vi "message_sendReply.vi"(0 "Host_Reference":refnum<class "HGF_Reference.lvclass">, 1 "MoAgSy_Message":refnum<class "MoAgSy_Message.lvclass">, 2 "timeout in ms (-1)":i32=-1, 5 "error in (no error)":errorcluster, 6 "Message":string, 8 "message":T1(ring), 9 "Message Type":enum16{"error Reply", "reply", "PublicKey"}(ring)) -> (14 "dup Host_Reference":refnum<class "HGF_Reference.lvclass">, 19 "error out":errorcluster)   [LabVIEW 2009, in "MoAgSy.lvlib" / "MoAgSy_Host.lvclass"]
doc: "<B>public</B> VI sends reply from referenced Host to an incoming message.\n<B> still in progress, only SV available</B>\n\nF.Berck@gsi.de\nGSI Darmstadt 2009"
uses:
  MoAgSy_Host.lvclass
  HGF_BaseClasses/HGF_Reference/HGF_Reference.lvclass
  MoAgSy_Message/MoAgSy_Message.lvclass
  MoAgSy_Factory/MoAgSy_Factory.lvclass
  HGF_BaseClasses/HGF_Factory/HGF_Factory.lvclass
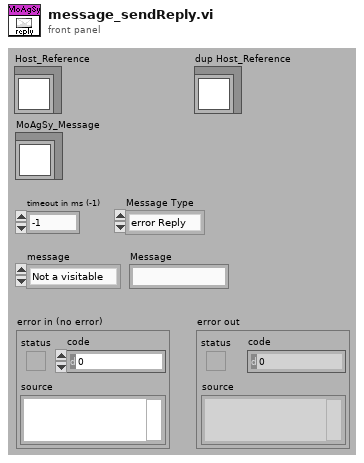
[diagram p1: front panel]
types:
  T1 = enum16{"Not a visitable", "Agent blacklisted", "Host full", "ok", "Class Unknown"}
  T2 = cluster{"Host Name":string, "Maximum number of running Agents":i16, "ID":string}
  T3 = cluster{"Host Variable":refnum<k21>, "Agent_Event (Monitor Event)":refnum<class "HGF_Event.lvclass">, "Host_Event (Monitor Event)":refnum<class "HGF_Event.lvclass">, "DSCException":refnum<class "HGF_TriggeredEvent.lvclass">, "MoAgSy_DSCThreadPool":refnum<class "HGF_Reference.lvclass">, "ManagerEvent":refnum<class "HGF_Event.lvclass">, "DSCDestination":refnum<class "HGF_TriggeredEvent.lvclass">}
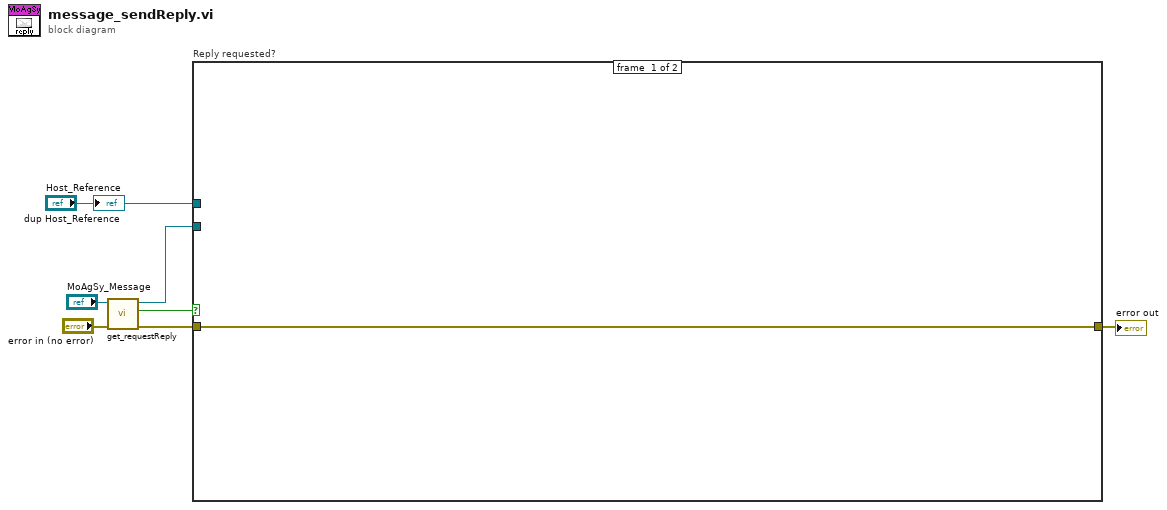
[diagram p0: block diagram]
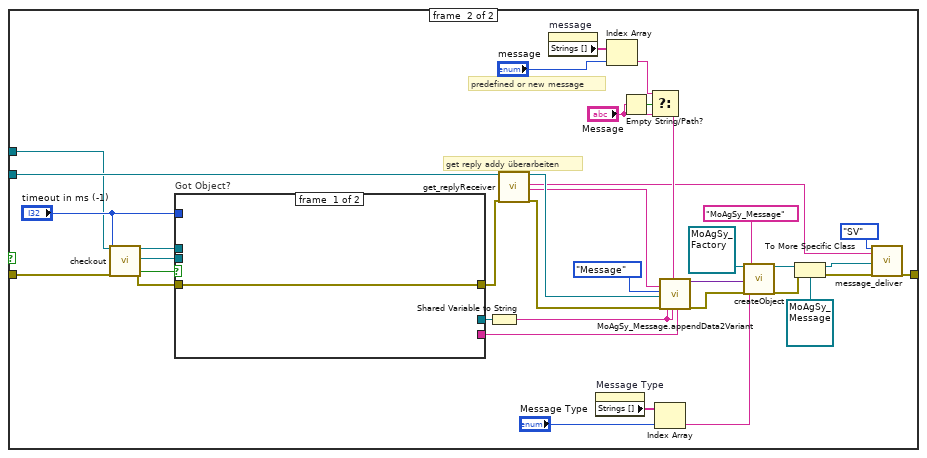
[diagram p2: hidden frame]
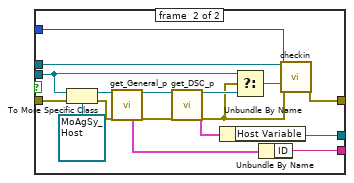
[diagram p3: hidden frame]
diagram:
  n1 = call "get_requestReply.vi"("error in (no error)"="error in (no error)", "MoAgSy_Message.lvclass in"="MoAgSy_Message") -> ("error out"=w2:errorcluster, "request reply"=w4:bool, "MoAgSy_Message.lvclass out"=w5:refnum<class "MoAgSy_Message.lvclass">)  [unwired: 7 out]
  n2 = case "Reply requested?" shown="True" w4 {
    tunnel: w5 -> [_ w35]
    tunnel: [w8 w18] -> w7
    tunnel: w2 -> [w8 w17]
    tunnel: "Host_Reference" -> [_ w16]
    frame #0 {
    }
    frame #1 {
      # "predefined or new message"
      # "get reply addy überarbeiten"
      n3 = call "checkout.vi"("HGF_Reference"=w16, "timeout in ms (-1)"="timeout in ms (-1)", "error in (no error)"=w17) -> ("dup HGF_Reference"=w41:refnum<class "HGF_Reference.lvclass">, "Object"=w43:refnum<class>, "got object?"=w42:bool, "error out"=w44:errorcluster)  [unwired: 13 out]
      n4 = case "Got Object?" shown="True" w42 {
        tunnel: w43 -> [_ w57]
        tunnel: w41 -> [_ w62]
        tunnel: "timeout in ms (-1)" -> [_ w61]
        tunnel: [w46 w60] -> w33
        tunnel: w44 -> [w46 w59]
        tunnel: [_ w55] -> w14
        tunnel: [_ w53] -> w24
        frame #0 {
        }
        frame #1 {
          n5 = To More Specific Class(target class=refnum<class "MoAgSy_Host.lvclass"> refnum ("MoAgSy.lvlib:MoAgSy_Host.lvclass"), reference=w57, error in=w59) -> (specific class reference=w52:refnum<class "MoAgSy_Host.lvclass">, error out=w50:errorcluster)
          n6 = call "get_General_p.vi"("MoAgSy_Host"=w52, "error in (no error)"=w50) -> ("dup MoAgSy_Host"=w48:refnum<class "MoAgSy_Host.lvclass">, "General"=w56:T2, "error out"=w49:errorcluster)  [unwired: 15 out]
          n7 = call "get_DSC_p.vi"("MoAgSy_Host"=w48, "error in (no error)"=w49) -> ("dup MoAgSy_Host"=w51:refnum<class "MoAgSy_Host.lvclass">, "DSC"=w54:T3, "error out"=w47:errorcluster)  [unwired: 15 out]
          n8 = Unbundle By Name(w54) -> ("Host Variable"=w53:refnum<k21>)
          n9 = Select(t=w57, s=w47, f=w51) -> (s? t:f=w58:refnum<class>)
          n10 = Unbundle By Name(w56) -> ("ID"=w55:string)
          n11 = call "checkin.vi"("HGF_Reference"=w62, "Object"=w58, "timeout /ms (-1)"=w61, "error in (no error)"=w47) -> ("error out"=w60:errorcluster)  [unwired: 15 out]
        }
      }
      n12 = Shared Variable to String(1:w24) -> (0:w15:string)
      n13 = call "get_replyReceiver.vi"("MoAgSy_Message"=w35, "error in (no error)"=w33) -> ("dup MoAgSy_Message"=w34:refnum<class "MoAgSy_Message.lvclass">, "reply to"=w9:string, "addressee"=w25:string, "error out"=w45:errorcluster)  [unwired: 14 out]
      n14 = property on="message" class="Enum (strict)"() -> ("Strings []"=w23:string[])  [unwired: 2 in, 2 out]
      n15 = property on="Message Type" class="Enum (strict)"() -> ("Strings []"=w21:string[])  [unwired: 2 in, 2 out]
      n16 = Index Array(array=w23, index="message") -> (element=w11:string)
      n17 = Empty String/Path?(string/path="Message") -> (empty?=w13:bool)
      n18 = Select(t=w11, s=w13, f="Message") -> (s? t:f=w10:string)
      n19 = Index Array(array=w21, index="Message Type") -> (element=w19:string)
      n20 = call "MoAgSy_Message.appendData2Variant.vi"("addressee"=w25, "type"=enum16{"mobile Agent", "Visitor", "Message"}."Message", "Object"=w34, "error in"=w45, "sender"=w15, "message"=w10, "reply to"=w15, "reply id"=w14) -> ("dup_initData"=w36:variant, "error out"=w32:errorcluster)  [unwired: 3 in, 7 out]
      n21 = call "createObject.vi"("HGF_Factory"=refnum<class "MoAgSy_Factory.lvclass"> refnum ("MoAgSy.lvlib:MoAgSy_Factory.lvclass"), "objectName"=w19, "initializationData"=w36, "error in (no error)"=w32, "className"="MoAgSy_Message") -> ("HGF_Object"=w31:refnum<class "HGF_Factory.lvclass">, "error out"=w30:errorcluster)  [unwired: 13 out]
      n22 = To More Specific Class(target class=refnum<class "MoAgSy_Message.lvclass"> refnum ("MoAgSy.lvlib:MoAgSy_Message.lvclass"), reference=w31, error in=w30) -> (specific class reference=w27:refnum<class "MoAgSy_Message.lvclass">, error out=w29:errorcluster)
      n23 = call "message_deliver.vi"("communication type"=enum16{"SV", "Dim"}."SV", "shared variable refnum"=w9, "MoAgSy_Message"=w27, "error in (no error)"=w29) -> ("error out"=w18:errorcluster)  [unwired: 15 out]
    }
  }
  "error out" <- w7
  "dup Host_Reference" <- "Host_Reference"
